vi "Email Purchase Report.vi"() -> ()   [LabVIEW 2010]
uses:
  <vilib>/Utility/file.llb/Read From Spreadsheet File (string).vi
  <vilib>/Utility/file.llb/Write To Spreadsheet File (string).vi
panel:
  in  "Filter Incoming Fundraiser Submissions?":bool=TRUE
  out "x-y*floor(x/y)":i32
  out "previous":string
  out "number of replacements":i32
  out "extension 2":string
  out "appended path 2":path
  out "Numeric 2":i32
  out "Totals String":string
  out "Email 2":string
  out "CC (Carbon Copy Recipient - Optional)":string="matthew.saverin@colorado.edu, logan.t.meyer@gmail.com"
  out "Sender's Email Address (eg: jsmith77@gmail.com)":string="logan.t.meyer@gmail.com"
  out "appended path":path
  out "Body":string
  out "Numeric":i32
  out "array w/ subset deleted 2":string[][](array[string])
  out "Item Info Text String":string
  out "Commission Percentage":string
  out "Commission ($)":string
  out "Website":string
  out "Product Price":string
  out "Product Name":string
  out "Email":string
  out "Last Name":string
  out "First Name":string
  out "Organization Name":string
  in  "Send Emails?":bool
  out "Array 2":string[](array[string])
  out "Array":string[](array[string])
  out "element":string
  out "array w/ subset deleted":string[][](array[string])
  in  "Empty Array":string[][](array[string])=[["Accuracy", "Extension", "Book Name", "Book Listing Price", "Number of Transactions", "Total Book Price", "Retailer", "Commission", "Commission Percentage"]]
  out "extension":string
  out "Total Effective Commission":dbl
  out "Total Sales":dbl
  out "mean total effective commission rate":dbl format="%0.2f"
  out "All relevant purchases to extension":string[][](array[string])
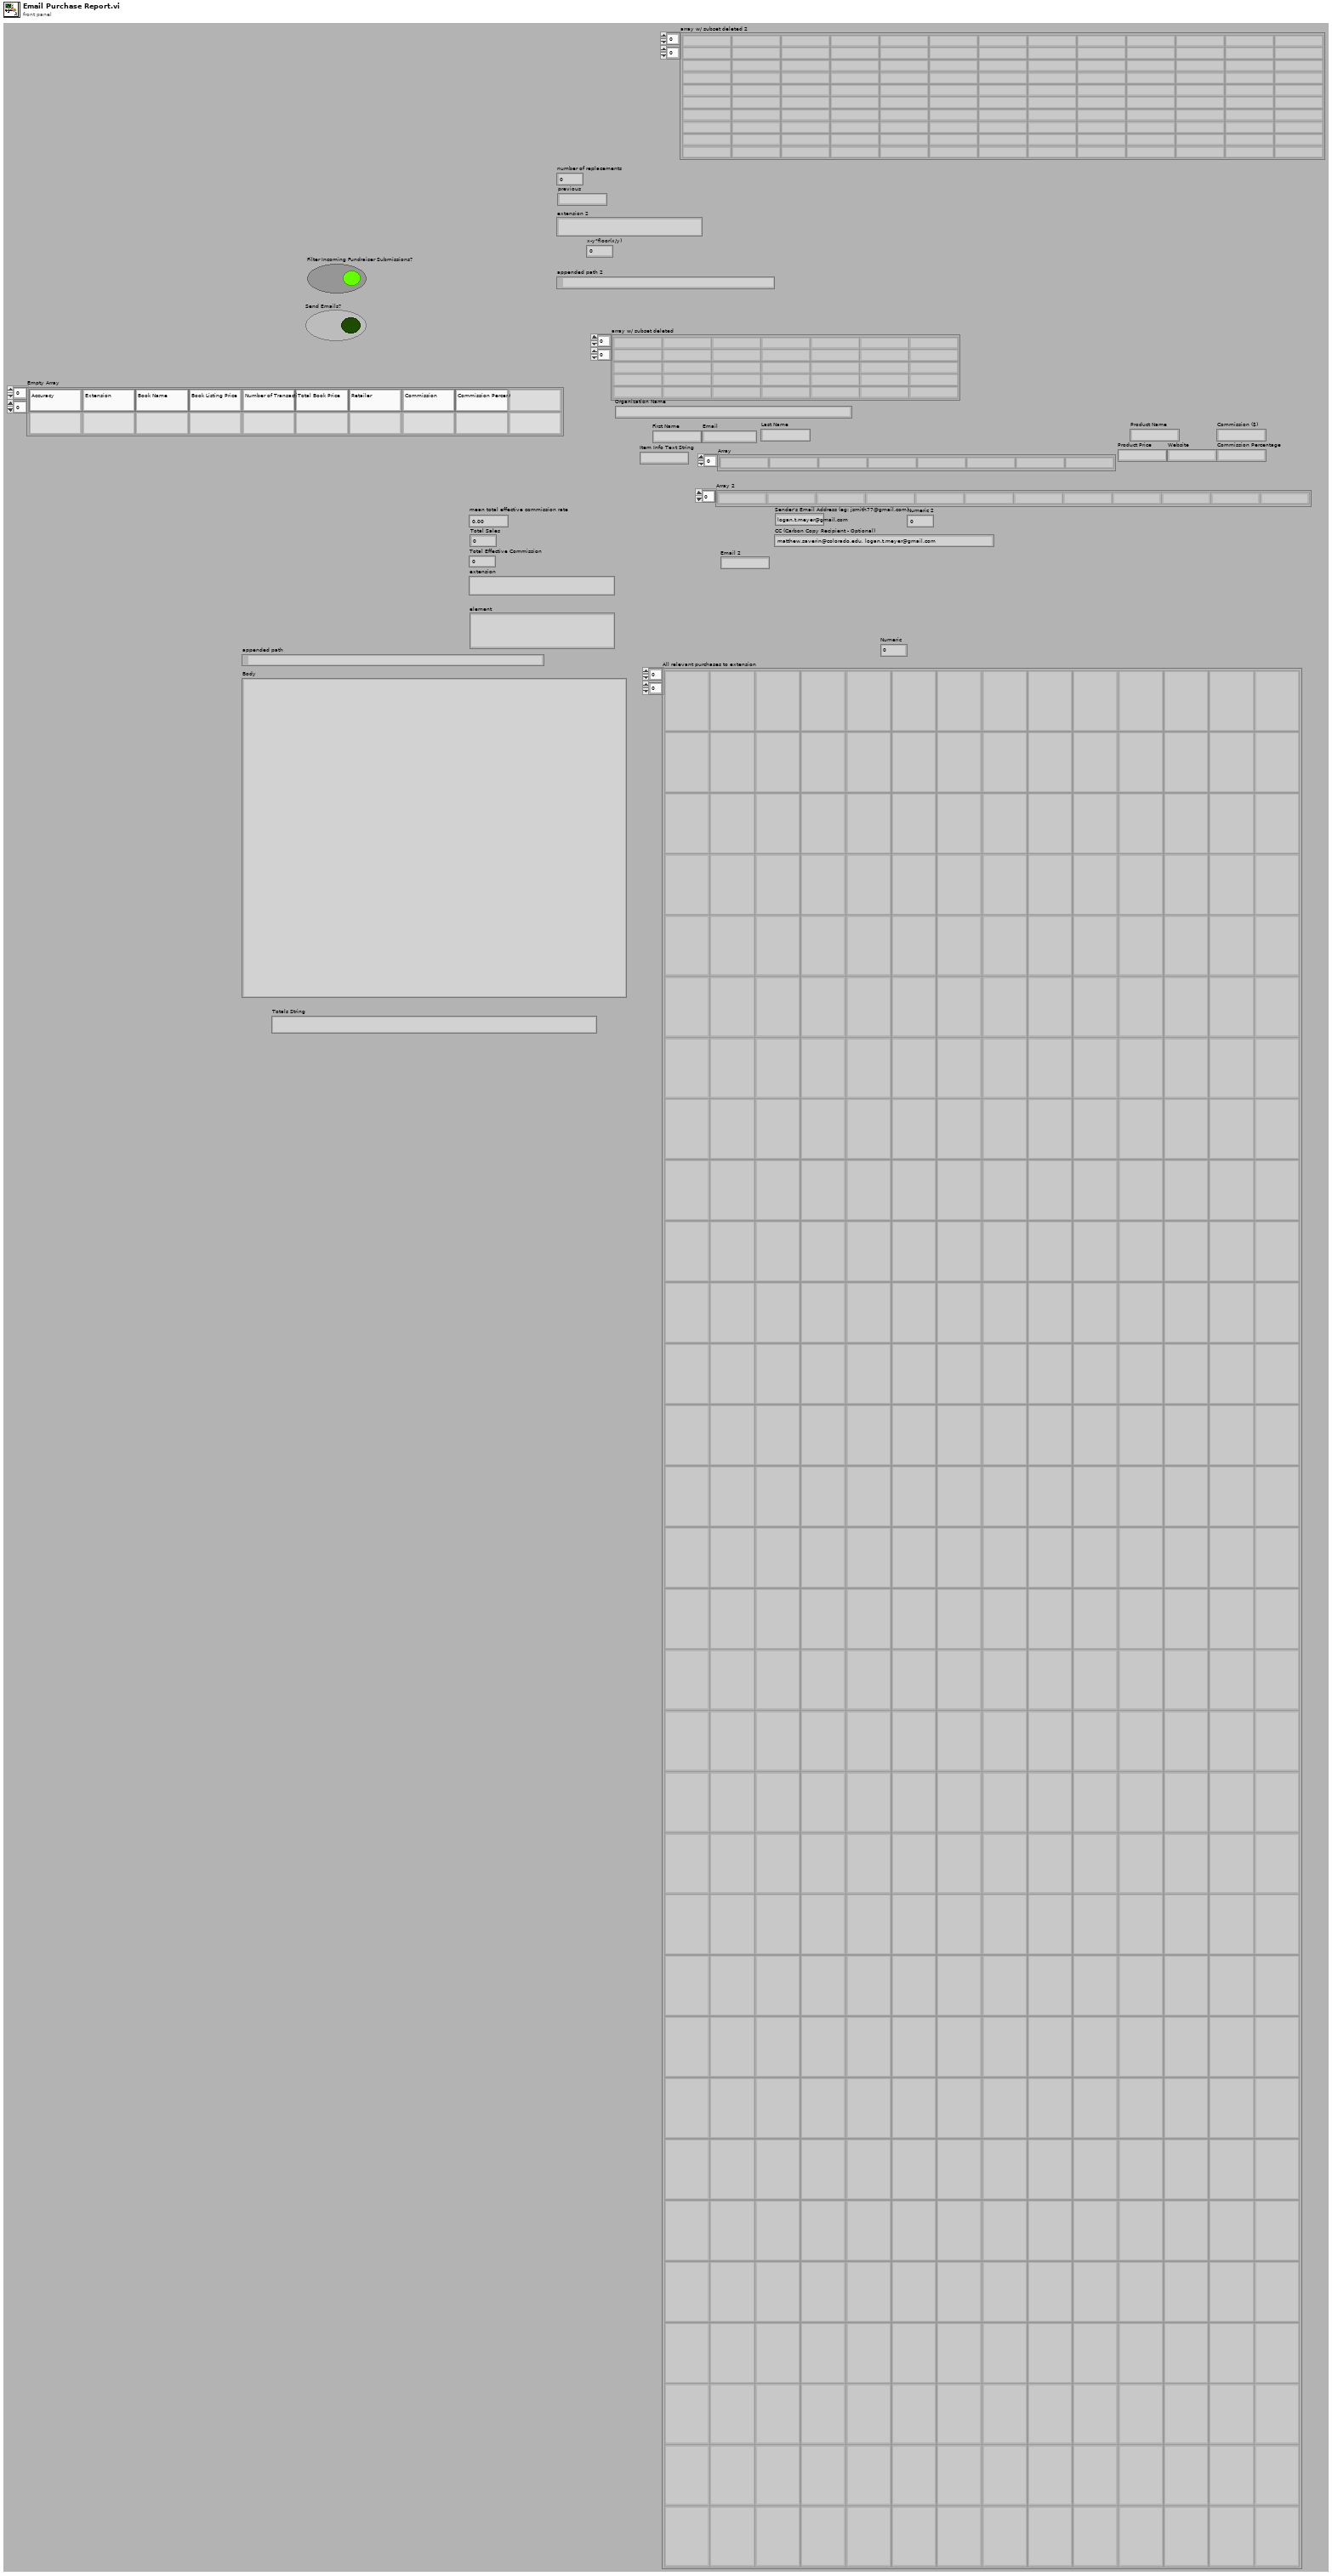
[diagram p1: front panel]
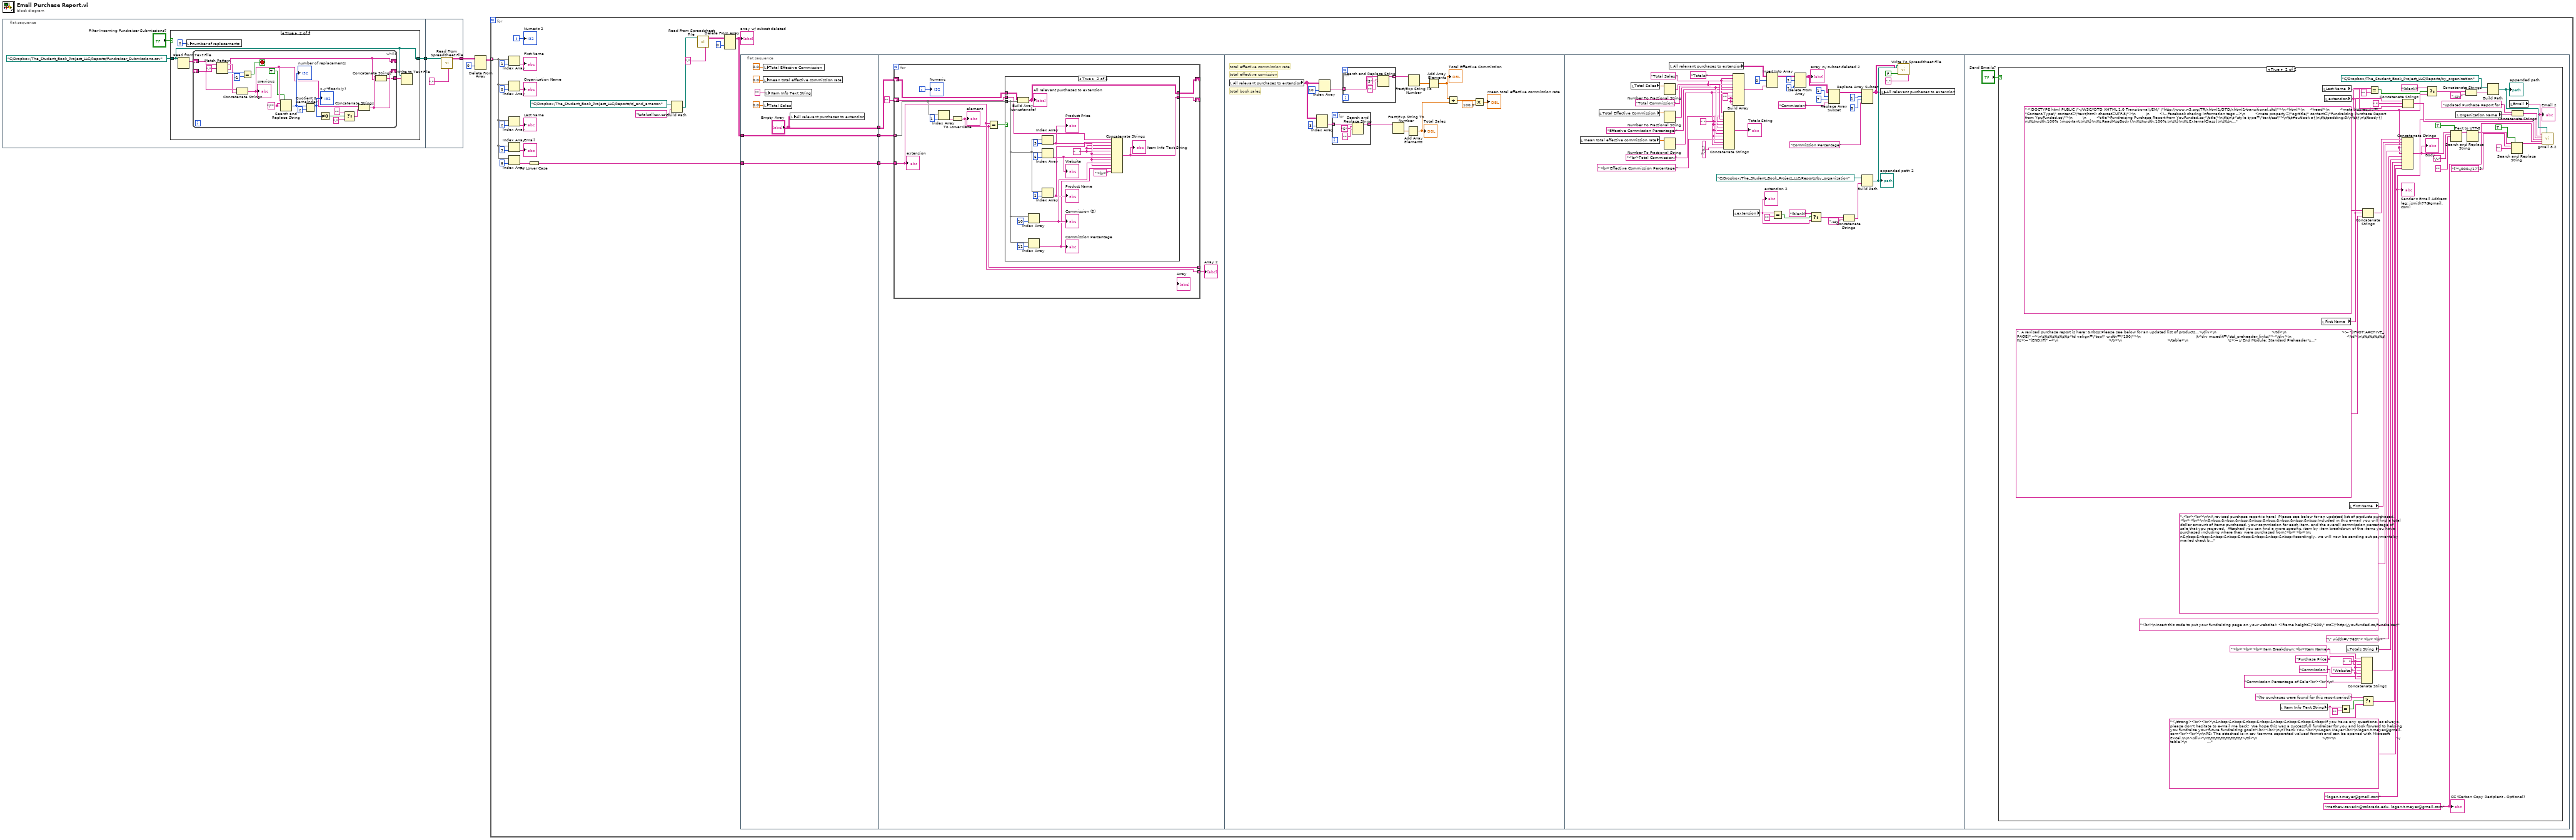
[diagram p0: block diagram]
diagram:
  n1 = flat-sequence {
    tunnel: [w7] -> w1
    tunnel: [w34] -> w2
    tunnel: w1 -> [w33]
    frame #0 {
      n2 = case shown="True" "Filter Incoming Fundraiser Submissions?" {
        tunnel: [w8 w9] -> w7
        tunnel: path "C:/Dropbox/The_Student_Book_Project_LLC/Reports/Fundraiser_Submissions.csv" ("file path (dialog if empty)") -> [w8 w9]
        frame False {
        }
        frame True {
          n3 = Read from Text File(file (use dialog)=w9) -> (text=w12:string)  [unwired: 3 in, 3 out]
          n4 = local write "number of replacements"(0 ("number of replacements")) -> ()
          n5 = while {
            shift-right: [w17] -> _
            shift-left: w12 -> [w32]
            shift-right: [w18] -> _
            shift-left: _ -> [w19]
            tunnel: [w16] -> w11
            stop <- w22 stop-if-true
            w25 = "\"" ("search string")
            n6 = Match Pattern(string=w32, regular expression=",") -> (before substring=w23:string, after substring=w17:string, offset past match=w30:i32)  [unwired: 1 in, 1 out]
            n7 = Concatenate Strings(w19, w23) -> (w20:string)
            "previous" <- w20
            n8 = Equal?(x=w30, y=-1) -> (x = y?=w22:bool)
            n9 = Search and Replace String(replace all?=TRUE ("replace all? (F)"), input string=w20, search string=w25, replace string=w25) -> (number of replacements=w26:i32)  [unwired: 4 in, 3 out]
            "number of replacements" <- w26
            n10 = Quotient & Remainder(x=w26, y=2) -> (x-y*floor(x/y)=w24:i32)  [unwired: 1 out]
            "x-y*floor(x/y)" <- w24
            n11 = Not Equal To 0?(x=w24) -> (x != 0?=w28:bool)
            n12 = Select(t="" ("search string"), s=w28, f=",") -> (s? t:f=w21:string)
            n13 = Concatenate Strings(w20, w21) -> (w18:string)
            n14 = Concatenate Strings(w18, w17) -> (w16:string)
          }
          n15 = Write to Text File(file (use dialog)=w9, text=w11) -> ()  [unwired: 2 in, 3 out]
        }
      }
    }
    frame #1 {
      n16 = call-poly <vilib>:"Read From Spreadsheet File.vi"("delimiter (\\t)"="," ("delimiter (\\t)"), "file path (dialog if empty)"=w33) -> ("all rows"=w34:string[][])  [unwired: 5 in, 4 out]
    }
  }
  n17 = Delete From Array(array=w2, index (row)=0) -> (array with subset deleted=w3:string[][])  [unwired: 2 in, 1 out]
  n18 = for {
    tunnel: w3 -> [w41] mode=indexing
    i -> [w36]
    n19 = Index Array(array=w41, index=1) -> (element=→"First Name":string)
    n20 = Index Array(array=w41, index=0) -> (element=→"Organization Name":string)
    n21 = Index Array(array=w41, index=2) -> (element=→"Last Name":string)
    n22 = Index Array(array=w41, index=3) -> (element=→"Email":string)
    n23 = Index Array(array=w41, index=6) -> (element=w37:string)
    n24 = To Lower Case(string=w37) -> (all lower case string=w47:string)
    n25 = Build Path(base path=path "C:/Dropbox/The_Student_Book_Project_LLC/Reports/cj_and_amazon" ("file path (dialog if empty)"), name or relative path="totalsallcsv.csv") -> (appended path=w53:path)
    n26 = call-poly <vilib>:"Read From Spreadsheet File.vi"("delimiter (\\t)"="," ("delimiter (\\t)"), "file path (dialog if empty)"=w53) -> ("all rows"=w56:string[][])  [unwired: 5 in, 4 out]
    n27 = Delete From Array(array=w56, index (row)=0) -> (array with subset deleted=w52:string[][])  [unwired: 2 in, 1 out]
    "array w/ subset deleted" <- w52
    n28 = flat-sequence {
      tunnel: w47 -> [w60]
      tunnel: w52 -> [w65]
      tunnel: [w65] -> w50
      tunnel: [w60] -> w49
      tunnel: ["Empty Array"] -> w48
      tunnel: w50 -> [w70]
      tunnel: w49 -> [w69]
      tunnel: w48 -> [w67]
      frame #0 {
        n29 = local write "Total Effective Commission"(0.0 ("Total Effective Commission")) -> ()
        n30 = local write "mean total effective commission rate"(0.0 ("mean total effective commission rate")) -> ()
        n31 = local write "Total Sales"(0.0 ("Total Book Sales")) -> ()
        n32 = local write "Item Info Text String"("" ("Book Info Text String")) -> ()
        n33 = local write "All relevant purchases to extension"("Empty Array") -> ()
      }
      frame #1 {
        n34 = for {
          tunnel: w70 -> [w79] mode=indexing
          tunnel: w69 -> [w78]
          tunnel: [w74] -> _ mode=indexing
          tunnel: [w78] -> w68 mode=indexing
          shift-right: [w76] -> _
          shift-left: w67 -> [w77]
          shift-right: [w72] -> _
          shift-left: "" -> [w73]
          i -> [w71]
          n35 = Index Array(array=w79, index=1) -> (element=w75:string)
          n36 = To Lower Case(string=w75) -> (all lower case string=w74:string)
          "element" <- w74
          n37 = Equal?(x=w78, y=w74) -> (x = y?=w80:bool)
          n38 = case shown="True" w80 {
            tunnel: w79 -> [_ w94]
            tunnel: w77 -> [w83 w100]
            tunnel: [w83 w84] -> w76
            tunnel: w73 -> [w82 w86]
            tunnel: [w82 w85] -> w72
            frame False {
            }
            frame True {
              w89 = "   " ("string")
              n39 = Build Array (concatenate)(w100, w94) -> (w84:string[][])
              "All relevant purchases to extension" <- w84
              n40 = Index Array(array=w94, index=10) -> (element=w90:string)
              "Commission ($)" <- w90
              n41 = Index Array(array=w94, index=11) -> (element=w88:string)
              "Commission Percentage" <- w88
              n42 = Index Array(array=w94, index=3) -> (element=w92:string)
              "Product Price" <- w92
              n43 = Index Array(array=w94, index=6) -> (element=w91:string)
              "Website" <- w91
              n44 = Index Array(array=w94, index=2) -> (element=w93:string)
              "Product Name" <- w93
              n45 = Concatenate Strings(w86, w93, w89, w89, w92, w89, w91, w89, w90, w89, w88, "<br>" ("string")) -> (w85:string)
              "Item Info Text String" <- w85
            }
          }
          "extension" <- w78
          "Numeric" <- w71
        }
        "Array 2" <- w68
      }
      frame #2 {
        # "total effective commission rate"
        # "total book sales"
        # "total effective comission"
        n46 = local read "All relevant purchases to extension"() -> (w110:string[][])
        n47 = Index Array(array=w110, index (col)=3 ("disabled index (col)")) -> (element=w104:string[])  [unwired: 1 in]
        n48 = Index Array(array=w110, index (col)=10 ("disabled index (col)")) -> (element=w102:string[])  [unwired: 1 in]
        n49 = for {
          tunnel: w104 -> [w120] mode=indexing
          tunnel: [w119] -> w103 mode=indexing
          n50 = Search and Replace String(input string=w120, search string="$", replace string="" ("replace string (\"\")")) -> (result string=w119:string)  [unwired: 5 in, 3 out]
        }
        n51 = for {
          tunnel: w102 -> [w116] mode=indexing
          tunnel: [w115] -> w101 mode=indexing
          n52 = Search and Replace String(input string=w116, search string="$", replace string="" ("replace string (\"\")")) -> (result string=w115:string)  [unwired: 5 in, 3 out]
        }
        n53 = Fract/Exp String To Number(string=w103) -> (number=w112:dbl[])  [unwired: 3 in, 1 out]
        n54 = Add Array Elements(numeric array=w112) -> (sum=w108:dbl)
        "Total Sales" <- w108
        n55 = Fract/Exp String To Number(string=w101) -> (number=w111:dbl[])  [unwired: 3 in, 1 out]
        n56 = Add Array Elements(numeric array=w111) -> (sum=w109:dbl)
        "Total Effective Commission" <- w109
        n57 = Divide(x=w109, y=w108) -> (x/y=w107:dbl)
        n58 = Multiply(x=w107, y=100.0) -> (x*y=→"mean total effective commission rate":dbl)
      }
      frame #3 {
        w138 = " " ("string")
        w162 = "" ("element")
        w125 = "Total Sales:" ("element")
        n59 = local read "mean total effective commission rate"() -> (w151:dbl)
        n60 = local read "Total Effective Commission"() -> (w152:dbl)
        n61 = local read "Total Sales"() -> (w153:dbl)
        n62 = Number To Fractional String(number=w153) -> (F-format string=w142:string)  [unwired: 3 in]
        n63 = Number To Fractional String(number=w152) -> (F-format string=w140:string)  [unwired: 3 in]
        n64 = Number To Fractional String(number=w151) -> (F-format string=w137:string)  [unwired: 3 in]
        n65 = local read "All relevant purchases to extension"() -> (w161:string[][])
        n66 = Concatenate Strings(w125, w138, w142, w138, w138, "<br>Total Commission:" ("element"), w138, w140, w138, "<br>Effective Commission Percentage:" ("element"), w138, w137, "\n\n" ("string")) -> (→"Totals String":string)
        n67 = Build Array("Totals:" ("name or relative path"), w125, w142, "Total Commission:" ("element"), w140, "Effective Commission Percentage:" ("element"), w137, w162, w162, w162, w162) -> (w163:string[])
        n68 = local read "extension"() -> (w148:string)
        "extension 2" <- w148
        n69 = Insert Into Array(array=w161, index (row)=0, new element=w163) -> (w145:string[][])  [unwired: 1 in]
        n70 = Equal?(x=w148, y="") -> (x = y?=w149:bool)
        n71 = Delete From Array(array=w145, length=3, index (col)=7 ("index (row)")) -> (array with subset deleted=w134:string[][])  [unwired: 1 in, 1 out]
        "array w/ subset deleted 2" <- w134
        n72 = Select(t="(blank)", s=w149, f=w148) -> (s? t:f=w146:string)
        n73 = Replace Array Subset(array=w134, new element="Commission" ("new element/subarray"), index (row)=1 ("disabled index (row)"), index (col)=7 ("disabled index (col)")) -> (w127:string[][])
        n74 = Concatenate Strings(w146, ".csv" ("string")) -> (w158:string)
        n75 = Replace Array Subset(array=w127, new element="Commission Percentage" ("new element/subarray"), index (row)=1 ("disabled index (row)"), index (col)=8 ("disabled index (col)")) -> (w126:string[][])
        n76 = Build Path(base path=path "C:/Dropbox/The_Student_Book_Project_LLC/Reports/by_organization" ("file path (dialog if empty)"), name or relative path=w158) -> (appended path=w156:path)
        "appended path 2" <- w156
        n77 = local write "All relevant purchases to extension"(w126) -> ()
        n78 = call-poly <vilib>:"Write To Spreadsheet File.vi"("delimiter (\\t)"="," ("delimiter (\\t)"), "append to file? (new file:F)"=FALSE, "2D data"=w126, "file path (dialog if empty)"=w156) -> ()  [unwired: 4 in, 1 out]
      }
      frame #4 {
        n79 = case shown="True" "Send Emails?" {
          frame False {
          }
          frame True {
            w213 = "   " ("string")
            w169 = "matthew.saverin@colorado.edu, logan.t.meyer@gmail.com" ("CC (Carbon Copy Recipient - Optional)")
            w190 = "logan.t.meyer@gmail.com" ("Sender's Email Address (eg: jsmith77@gmail.com)")
            n80 = local read "Item Info Text String"() -> (w172:string)
            n81 = local read "First Name"() -> (w188:string)
            n82 = local read "Last Name"() -> (w197:string)
            n83 = local read "extension"() -> (w167:string)
            n84 = Equal?(x=w172, y="") -> (x = y?=w174:bool)
            n85 = local read "Totals String"() -> (w198:string)
            n86 = local read "First Name"() -> (w214:string)
            n87 = Concatenate Strings("<br><br><br>Item Breakdown:<br>Item Name," ("string"), w213, "Purchase Price," ("string"), w213, "Website," ("string"), w213, "Commission," ("string"), w213, "Commission Percentage of Sale<br><br>\n" ("string")) -> (w207:string)
            n88 = Concatenate Strings("<!DOCTYPE html PUBLIC \"-//W3C//DTD XHTML 1.0 Transitional//EN\" \"http://www.w3.org/TR/xhtml1/DTD/xhtml1-transitional.dtd\">\n<html>\n    <head>\n        <meta http-equiv=\"Content-Type\" content=\"text/html; charset=UTF-8\">\n        \n        <!-- Facebook sharing information tags -->\n        <meta property=\"og:title\" content=\"Fundraising Purchase Report from YouFunded.co\">\n        \n        <title>Fundraising Purchase Report from YouFunded.co</title>\n\t\t\n\t<style type=\"text/css\">\n\t\t#outlook a{\n\t\t\tpadding:0;\n\t\t}\n\t\tbody{\n\t\t\twidth:100% !important;\n\t\t}\n\t\t.ReadMsgBody{\n\t\t\twidth:100%;\n\t\t}\n\t\t.ExternalClass{\n\t\t\twidth:100%;\n\t\t}\n\t\tbody{\n\t\t\t-webkit-text-size-adjust:none;\n\t\t}\n\t\tbody{\n\t\t\tmargin:0;\n\t\t\tpadding:0;\n\t\t}\n\t\timg{\n\t\t\tborder:0;\n\t\t\theight:auto;\n\t\t\tline-height:100%;\n\t\t\toutline:none;\n\t\t\ttext-decoration:none;\n\t\t}\n\t\ttable td{\n\t\t\tborder-collapse:collapse;\n\t\t}\n\t\t#backgroundTable{\n\t\t\theight:100% !important;\n\t\t\tmargin:0;\n\t\t\tpadding:0;\n\t\t\twidth:100% !important;\n\t\t}\n\t/*\n\t@tab Page\n\t@section background color\n\t@tip Set the background color for your email. You may want to choose one that matches your company's branding.\n\t@theme page\n\t*/\n\t\tbody,#backgroundTable{\n\t\t\t/*@editable*/background-color:#fafafa;\n\t\t}\n\t/*\n\t@tab Page\n\t@section email border\n\t@tip Set the border for your email.\n\t*/\n\t\t#templateContainer{\n\t\t\t/*@editable*/border:1px solid #DDDDDD;\n\t\t}\n\t/*\n\t@tab Page\n\t@section heading 1\n\t@tip Set the styling for all first-level headings in your emails. These should be the largest of your headings.\n\t@style heading 1\n\t*/\n\t\th1,.h1{\n\t\t\t/*@editable*/color:#202020;\n\t\t\tdisplay:block;\n\t\t\t/*@editable*/font-family:Arial;\n\t\t\t/*@editable*/font-size:34px;\n\t\t\t/*@editable*/font-weight:bold;\n\t\t\t/*@editable*/line-height:100%;\n\t\t\tmargin-top:0;\n\t\t\tmargin-right:0;\n\t\t\tmargin-bottom:10px;\n\t\t\tmargin-left:0;\n\t\t\t/*@editable*/text-align:left;\n\t\t}\n\t/*\n\t@tab Page\n\t@section heading 2\n\t@tip Set the styling for all second-level headings in your emails.\n\t@style heading 2\n\t*/\n\t\th2,.h2{\n\t\t\t/*@editable*/color:#202020;\n\t\t\tdisplay:block;\n\t\t\t/*@editable*/font-family:Arial;\n\t\t\t/*@editable*/font-size:30px;\n\t\t\t/*@editable*/font-weight:bold;\n\t\t\t/*@editable*/line-height:100%;\n\t\t\tmargin-top:0;\n\t\t\tmargin-right:0;\n\t\t\tmargin-bottom:10px;\n\t\t\tmargin-left:0;\n\t\t\t/*@editable*/text-align:left;\n\t\t}\n\t/*\n\t@tab Page\n\t@section heading 3\n\t@tip Set the styling for all third-level headings in your emails.\n\t@style heading 3\n\t*/\n\t\th3,.h3{\n\t\t\t/*@editable*/color:#202020;\n\t\t\tdisplay:block;\n\t\t\t/*@editable*/font-family:Arial;\n\t\t\t/*@editable*/font-size:26px;\n\t\t\t/*@editable*/font-weight:bold;\n\t\t\t/*@editable*/line-height:100%;\n\t\t\tmargin-top:0;\n\t\t\tmargin-right:0;\n\t\t\tmargin-bottom:10px;\n\t\t\tmargin-left:0;\n\t\t\t/*@editable*/text-align:left;\n\t\t}\n\t/*\n\t@tab Page\n\t@section heading 4\n\t@tip Set the styling for all fourth-level headings in your emails. These should be the smallest of your headings.\n\t@style heading 4\n\t*/\n\t\th4,.h4{\n\t\t\t/*@editable*/color:#202020;\n\t\t\tdisplay:block;\n\t\t\t/*@editable*/font-family:Arial;\n\t\t\t/*@editable*/font-size:22px;\n\t\t\t/*@editable*/font-weight:bold;\n\t\t\t/*@editable*/line-height:100%;\n\t\t\tmargin-top:0;\n\t\t\tmargin-right:0;\n\t\t\tmargin-bottom:10px;\n\t\t\tmargin-left:0;\n\t\t\t/*@editable*/text-align:left;\n\t\t}\n\t/*\n\t@tab Header\n\t@section preheader style\n\t@tip Set the background color for your email's preheader area.\n\t@theme page\n\t*/\n\t\t#templatePreheader{\n\t\t\t/*@editable*/background-color:#FAFAFA;\n\t\t}\n\t/*\n\t@tab Header\n\t@section preheader text\n\t@tip Set the styling for your email's preheader text. Choose a size and color that is easy to read.\n\t*/\n\t\t.preheaderContent div{\n\t\t\t/*@editable*/color:#505050;\n\t\t\t/*@editable*/font-family:Arial;\n\t\t\t/*@editable*/font-size:10px;\n\t\t\t/*@editable*/line-height:100%;\n\t\t\t/*@editable*/text-align:left;\n\t\t}\n\t/*\n\t@tab Header\n\t@section preheader link\n\t@tip Set the styling for your email's preheader links. Choose a color that helps them stand out from your text.\n\t*/\n\t\t.preheaderContent div a:link,.preheaderContent div a:visited,.preheaderContent div a .yshortcuts {\n\t\t\t/*@editable*/color:#336699;\n\t\t\t/*@editable*/font-weight:normal;\n\t\t\t/*@editable*/text-decoration:underline;\n\t\t}\n\t/*\n\t@tab Header\n\t@section header style\n\t@tip Set the background color and border for your email's header area.\n\t@theme header\n\t*/\n\t\t#templateHeader{\n\t\t\t/*@editable*/background-color:#FFFFFF;\n\t\t\t/*@editable*/border-bottom:0;\n\t\t}\n\t/*\n\t@tab Header\n\t@section header text\n\t@tip Set the styling for your email's header text. Choose a size and color that is easy to read.\n\t*/\n\t\t.headerContent{\n\t\t\t/*@editable*/color:#202020;\n\t\t\t/*@editable*/font-family:Arial;\n\t\t\t/*@editable*/font-size:34px;\n\t\t\t/*@editable*/font-weight:bold;\n\t\t\t/*@editable*/line-height:100%;\n\t\t\t/*@editable*/padding:0;\n\t\t\t/*@editable*/text-align:center;\n\t\t\t/*@editable*/vertical-align:middle;\n\t\t}\n\t/*\n\t@tab Header\n\t@section header link\n\t@tip Set the styling for your email's header links. Choose a color that helps them stand out from your text.\n\t*/\n\t\t.headerContent a:link,.headerContent a:visited,.headerContent a .yshortcuts {\n\t\t\t/*@editable*/color:#336699;\n\t\t\t/*@editable*/font-weight:normal;\n\t\t\t/*@editable*/text-decoration:underline;\n\t\t}\n\t\t#headerImage{\n\t\t\theight:auto;\n\t\t\tmax-width:600px !important;\n\t\t}\n\t/*\n\t@tab Body\n\t@section body style\n\t@tip Set the background color for your email's body area.\n\t*/\n\t\t#templateContainer,.bodyContent{\n\t\t\t/*@editable*/background-color:#FFFFFF;\n\t\t}\n\t/*\n\t@tab Body\n\t@section body text\n\t@tip Set the styling for your email's main content text. Choose a size and color that is easy to read.\n\t@theme main\n\t*/\n\t\t.bodyContent div{\n\t\t\t/*@editable*/color:#505050;\n\t\t\t/*@editable*/font-family:Arial;\n\t\t\t/*@editable*/font-size:14px;\n\t\t\t/*@editable*/line-height:150%;\n\t\t\t/*@editable*/text-align:left;\n\t\t}\n\t/*\n\t@tab Body\n\t@section body link\n\t@tip Set the styling for your email's main content links. Choose a color that helps them stand out from your text.\n\t*/\n\t\t.bodyContent div a:link,.bodyContent div a:visited,.bodyContent div a .yshortcuts {\n\t\t\t/*@editable*/color:#336699;\n\t\t\t/*@editable*/font-weight:normal;\n\t\t\t/*@editable*/text-decoration:underline;\n\t\t}\n\t\t.bodyContent img{\n\t\t\tdisplay:inline;\n\t\t\theight:auto;\n\t\t}\n\t/*\n\t@tab Footer\n\t@section footer style\n\t@tip Set the background color and top border for your email's footer area.\n\t@theme footer\n\t*/\n\t\t#templateFooter{\n\t\t\t/*@editable*/background-color:#FFFFFF;\n\t\t\t/*@editable*/border-top:0;\n\t\t}\n\t/*\n\t@tab Footer\n\t@section footer text\n\t@tip Set the styling for your email's footer text. Choose a size and color that is easy to read.\n\t@theme footer\n\t*/\n\t\t.footerContent div{\n\t\t\t/*@editable*/color:#707070;\n\t\t\t/*@editable*/font-family:Arial;\n\t\t\t/*@editable*/font-size:12px;\n\t\t\t/*@editable*/line-height:125%;\n\t\t\t/*@editable*/text-align:left;\n\t\t}\n\t/*\n\t@tab Footer\n\t@section footer link\n\t@tip Set the styling for your email's footer links. Choose a color that helps them stand out from your text.\n\t*/\n\t\t.footerContent div a:link,.footerContent div a:visited,.footerContent div a .yshortcuts {\n\t\t\t/*@editable*/color:#336699;\n\t\t\t/*@editable*/font-weight:normal;\n\t\t\t/*@editable*/text-decoration:underline;\n\t\t}\n\t\t.footerContent img{\n\t\t\tdisplay:inline;\n\t\t}\n\t/*\n\t@tab Footer\n\t@section social bar style\n\t@tip Set the background color and border for your email's footer social bar.\n\t@theme footer\n\t*/\n\t\t#social{\n\t\t\t/*@editable*/background-color:#FAFAFA;\n\t\t\t/*@editable*/border:0;\n\t\t}\n\t/*\n\t@tab Footer\n\t@section social bar style\n\t@tip Set the background color and border for your email's footer social bar.\n\t*/\n\t\t#social div{\n\t\t\t/*@editable*/text-align:center;\n\t\t}\n\t/*\n\t@tab Footer\n\t@section utility bar style\n\t@tip Set the background color and border for your email's footer utility bar.\n\t@theme footer\n\t*/\n\t\t#utility{\n\t\t\t/*@editable*/background-color:#FFFFFF;\n\t\t\t/*@editable*/border:0;\n\t\t}\n\t/*\n\t@tab Footer\n\t@section utility bar style\n\t@tip Set the background color and border for your email's footer utility bar.\n\t*/\n\t\t#utility div{\n\t\t\t/*@editable*/text-align:center;\n\t\t}\n\t\t#monkeyRewards img{\n\t\t\tmax-width:190px;\n\t\t}\n</style></head>\n    <body leftmargin=\"0\" marginwidth=\"0\" topmargin=\"0\" marginheight=\"0\" offset=\"0\">\n    \t<center>\n        \t<table border=\"0\" cellpadding=\"0\" cellspacing=\"0\" height=\"100%\" width=\"100%\" id=\"backgroundTable\">\n            \t<tr>\n                \t<td align=\"center\" valign=\"top\">\n                        <!-- // Begin Template Preheader \\\\ -->\n                        <table border=\"0\" cellpadding=\"10\" cellspacing=\"0\" width=\"600\" id=\"templatePreheader\">\n                            <tr>\n                                <td valign=\"top\" class=\"preheaderContent\">\n                                \n                                \t<!-- // Begin Module: Standard Preheader \\ -->\n                                    <table border=\"0\" cellpadding=\"10\" cellspacing=\"0\" width=\"100%\">\n                                    \t<tr>\n                                        \t<td valign=\"top\">\n                                            \t<div mc:edit=\"std_preheader_content\">Hello " ("string"), w188, ", A revised purchase report is here! &nbsp;Please see below for an updated list of products...</div>\n                                            </td>\n                                            <!-- *|IFNOT:ARCHIVE_PAGE|* -->\n\t\t\t\t\t\t\t\t\t\t\t<td valign=\"top\" width=\"190\">\n                                            \t<div mc:edit=\"std_preheader_links\"></div>\n                                            </td>\n\t\t\t\t\t\t\t\t\t\t\t<!-- *|END:IF|* -->\n                                        </tr>\n                                    </table>\n                                \t<!-- // End Module: Standard Preheader \\ -->\n                                \n                                </td>\n                            </tr>\n                        </table>\n                        <!-- // End Template Preheader \\\\ -->\n                    \t<table border=\"0\" cellpadding=\"0\" cellspacing=\"0\" width=\"600\" id=\"templateContainer\">\n                        \t<tr>\n                            \t<td align=\"center\" valign=\"top\">\n                                    <!-- // Begin Template Header \\\\ -->\n                                \t<table border=\"0\" cellpadding=\"0\" cellspacing=\"0\" width=\"600\" id=\"templateHeader\">\n                                        <tr>\n                                            <td class=\"headerContent\">\n                                            \n                                            \t<!-- // Begin Module: Standard Header Image \\\\ -->\n                                            \t<img src=\"http://gallery.mailchimp.com/7b76da0200b336552015a7358/images/youfunded_purchse_report2.fwb1d1135f018387a6f7.png\" style=\"max-width:600px;\" id=\"headerImage campaign-icon\" mc:label=\"header_image\" mc:edit=\"header_image\" mc:allowdesigner mc:allowtext>\n                                            \t<!-- // End Module: Standard Header Image \\\\ -->\n                                            \n                                            </td>\n                                        </tr>\n                                    </table>\n                                    <!-- // End Template Header \\\\ -->\n                                </td>\n                            </tr>\n                        \t<tr>\n                            \t<td align=\"center\" valign=\"top\">\n                                    <!-- // Begin Template Body \\\\ -->\n                                \t<table border=\"0\" cellpadding=\"0\" cellspacing=\"0\" width=\"600\" id=\"templateBody\">\n                                    \t<tr>\n                                            <td valign=\"top\" class=\"bodyContent\">\n                                \n                                                <!-- // Begin Module: Standard Content \\\\ -->\n                                                <table border=\"0\" cellpadding=\"20\" cellspacing=\"0\" width=\"100%\">\n                                                    <tr>\n                                                        <td valign=\"top\">\n                                                            <div mc:edit=\"std_content00\"><h1 class=\"h1\" style=\"text-align: center;\">\n\tRevised Purchase Report</h1>\n<div style=\"text-align: center;\">\n\t&nbsp;</div>\n<div style=\"text-align: left;\">\nHello " ("string")) -> (w176:string)
            n89 = Select(t="(No purchases were found for this report period)", s=w174, f=w172) -> (s? t:f=w171:string)
            n90 = Equal?(x=w167, y="") -> (x = y?=w201:bool)
            n91 = Concatenate Strings(w176, w214, ",<br><br>\n\nA revised purchase report is here!  Please see below for an updated list of products purchased.<br><br>\n\n&nbsp;&nbsp;&nbsp;&nbsp;&nbsp;&nbsp;&nbsp;&nbsp;Included in this e-mail you will find a total dollar amount of items purchased, your commission for each item, and the overall commission percentage of sale that you recieved.  Attached you can find a more specific, item by item breakdown of the items you have purchased including where they were purchased from!<br><br>\n\n&nbsp;&nbsp;&nbsp;&nbsp;&nbsp;&nbsp;&nbsp;&nbsp;Accordingly, we will now be sending out payments by mailed check by March 8th, so if you have not provided us with your mailing address and information on who to make the payment out to, please reply to this email with you information so that we can make sure that the payment reaches you!<br><br>\n\n<strong>Your Purchase Report:<br><br>\n\nstatic fundraising page location: http://youfunded.co/" ("Body"), w167, "<br>\nInsert this code to put your fundraising page on your website!: <iframe height=\"600\" src=\"http://youfunded.co/Fundraiser/" ("string"), w167, "\" width=\"760\"><br><br>" ("string"), w198, w207, w171, "</strong><br><br>\n&nbsp;&nbsp;&nbsp;&nbsp;&nbsp;&nbsp;&nbsp;&nbsp;If you have any questions, as always, please don't hesitate to e-mail me back!  We hope this was a successfull fundraiser for you and look forward to helping you fundraise your future fundraising goals!<br><br>\n\nThank You,<br>\nLogan Meyer<br>\nlogan.t.meyer@gmail.com<br><br>\n\nPS: The attached is in csv (comma separated values) format and can be opened with Microsoft Excel.\n\n</div>\n\t\t\t\t\t\t\t\t\t\t\t\t\t\t</td>\n                                                    </tr>\n                                                </table>\n                                                <!-- // End Module: Standard Content \\\\ -->\n                                                \n                                            </td>\n                                        </tr>\n                                    </table>\n                                    <!-- // End Template Body \\\\ -->\n                                </td>\n                            </tr>\n                        \t<tr>\n                            \t<td align=\"center\" valign=\"top\">\n                                    <!-- // Begin Template Footer \\\\ -->\n                                \t<table border=\"0\" cellpadding=\"10\" cellspacing=\"0\" width=\"600\" id=\"templateFooter\">\n                                    \t<tr>\n                                        \t<td valign=\"top\" class=\"footerContent\">\n                                            \n                                                <!-- // Begin Module: Standard Footer \\\\ -->\n                                                <table border=\"0\" cellpadding=\"10\" cellspacing=\"0\" width=\"100%\">\n                                                    <tr>\n                                                        <td valign=\"middle\" id=\"social\">\n                                                            <div style=\"text-align: center;\" mc:edit=\"std_social\">&nbsp;<a href=\"https://twitter.com/YouFunded\" target=\"_self\">Follow on Twitter</a> | <a href=\"http://www.facebook.com/YouFunded\" target=\"_self\">Friend on Facebook</a></div>\n                                                        </td>\n                                                    </tr>\n                                                    <tr>\n                                                        <td valign=\"top\">\n                                                            <div mc:edit=\"std_footer\"><div style=\"text-align: center;\">\n\t<em>Copyright &copy; 2013 You Funded, All rights reserved.</em><br>\n\t<br>\n\t<strong>Any Questions? Please e-mail us at:</strong><br>\n\tLogan Meyer<br>\n\tlogan@youfunded.co<br>\n\tCommunity Team Member<br>\n\t<br>\n\tYouFunded.co</div>\n</div>\n                                                        </td>\n                                                  \n                                                </tr>\n                                               \n                                                </table>\n                                                <!-- // End Module: Standard Footer \\\\ -->\n                                            \n                                            </td>\n                                        </tr>\n                                    </table>\n                                    <!-- // End Template Footer \\\\ -->\n                                </td>\n                            </tr>\n                        </table>\n                        <br>\n                    </td>\n                </tr>\n            </table>\n        </center>\n    </body>\n</html>" ("string")) -> (w185:string)
            "Body" <- w185
            n92 = Concatenate Strings(w188, " " ("string"), w197) -> (w195:string)
            n93 = Select(t="(blank)", s=w201, f=w167) -> (s? t:f=w199:string)
            n94 = Search and Replace String(replace all?=TRUE ("replace all? (F)"), input string=w185, search string="/v", replace string="" ("replace string (\"\")")) -> (result string=w178:string)  [unwired: 4 in, 3 out]
            n95 = local read "Organization Name"() -> (w193:string)
            n96 = Concatenate Strings(w199, ".csv" ("string")) -> (w203:string)
            n97 = Text to UTF-8(11:w178) -> (3:w181:string)  [unwired: 1 in, 1 out]
            n98 = Build Path(base path=path "C:/Dropbox/The_Student_Book_Project_LLC/Reports/by_organization" ("file path (dialog if empty)"), name or relative path=w203) -> (appended path=w194:path)
            "appended path" <- w194
            n99 = local read "Email"() -> (w170:string)
            "Email 2" <- w170
            n100 = Search and Replace String(replace all?=TRUE ("replace all? (F)"), input string=w181, search string="[^\\000-\\177]", replace string="" ("replace string (\"\")")) -> (result string=w177:string)  [unwired: 4 in, 3 out]
            n101 = Concatenate Strings("Updated Purchase Report for " ("string"), w193) -> (w191:string)
            n102 = call "gmail 8.2.vi"("Recipient's Email Address Address"=w170, "Subject"=w191, "Sender's Email Address (eg: jsmith77@gmail.com)"=w190, "Recipient's Name"=w195, "CC (Carbon Copy Recipient - Optional)"=w169, "Body"=w177, "Attachment - Optional"=w194) -> ()  [unwired: 13 in]
            "Sender's Email Address (eg: jsmith77@gmail.com)" <- w190
            "CC (Carbon Copy Recipient - Optional)" <- w169
          }
        }
      }
    }
    "Numeric 2" <- w36
  }
